vi "SRV_Read Motors Config File.vi"(0 "Motors Config File Path":path, 11 "error in (no error)":errorcluster) -> (4 "Motors Config File Path out":path, 8 "Motor Control Config":T1[](array[typedef]) {"Release Cmds"."Motor Control Commands Array"."Value" format="%02x"; "Release Cmds"."Motor Control Commands Array"."Register" format="%02x"; "Release Cmds"."Motor Control Commands Array"."I2C Address" format="%02x"; "Press Cmds"."Motor Control Commands Array"."Value" format="%02x"; "Press Cmds"."Motor Control Commands Array"."Register" format="%02x"; "Press Cmds"."Motor Control Commands Array"."I2C Address" format="%02x"}, 10 "Cancelled?":bool, 15 "error out":errorcluster)   [LabVIEW 2014]
doc: "Author: Mike Schultz (LogicPD, Inc)"
uses:
  SRV_Motor Control Button Config.ctl
  SRV_Motor Legos-Servo.ctl
  SRV_Motor Control Commands Cluster.ctl
  SRV_Motor Control Command Config.ctl
  SRV_Motor Control Button Icons_FALSE.ctl
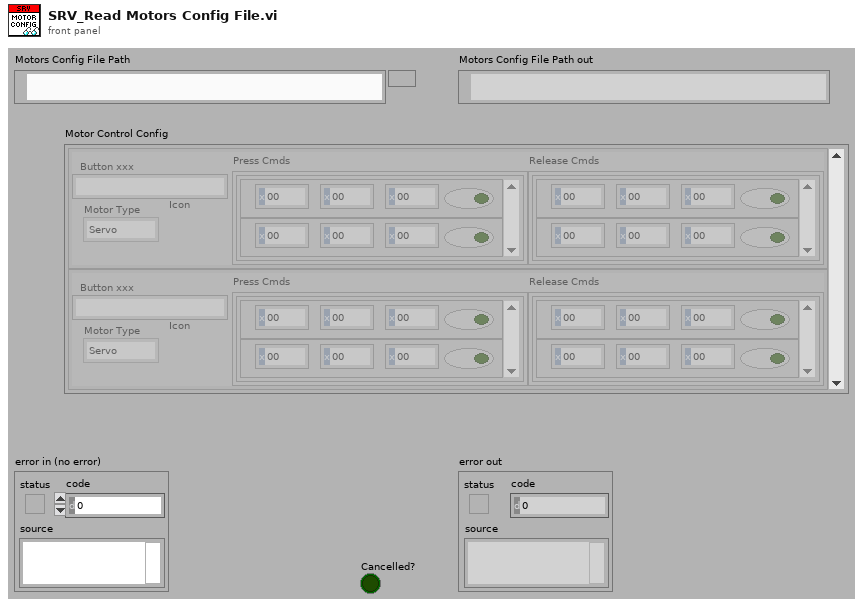
[diagram p1: front panel]
types:
  T1 = typedef "SRV_Motor Control Button Config.ctl" = cluster{"Button Name":string, "Button Label":string, "Motor Type":T2, "Press Cmds":T3, "Release Cmds":T3, "Icon":T5}
  T2 = typedef "SRV_Motor Legos-Servo.ctl" = enum16{"Servo", "Legos", "Shared Var"}
  T3 = typedef "SRV_Motor Control Commands Cluster.ctl" = cluster{"Motor Control Commands Array":T4[]}
  T4 = typedef "SRV_Motor Control Command Config.ctl" = cluster{"I2C Address":u8, "Register":u8, "Value":u8, "Active":bool}
  T5 = typedef "SRV_Motor Control Button Icons_FALSE.ctl" = u16
  T6 = enum16{"open", "open or create", "create or replace", "create", "open (read only)"}
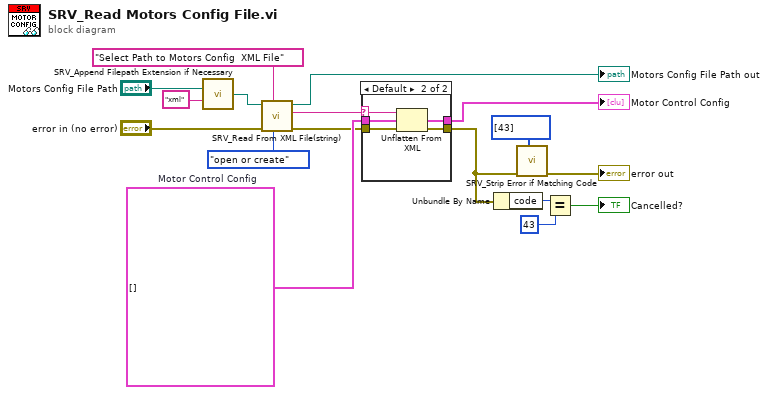
[diagram p0: block diagram]
diagram:
  w17 = T1[] []  # Motor Control Config
  n1 = call "SRV_Append Filepath Extension if Necessary.vi"("Filepath"="Motors Config File Path", "Extension"="xml") -> ("Filepath with Extension"=w11:path)  [unwired: 13 in]
  n2 = call "SRV_Read From XML File(string).vi"("function (open-read-only:4)"=T6."open or create", "Prompt"="Select Path to Motors Config  XML File", "error in (no error)"="error in (no error)", "XML File Path"=w11) -> ("error out"=w13:errorcluster, "XML Elements"=w9:string, "XML File Path(duplicate)"=→"Motors Config File Path out":path)  [unwired: 5 in]
  n3 = case shown="Default" w9 {
    selector: w9 -> [_ w20]
    tunnel: w17 -> [w18 w24]
    tunnel: [w18 w23] -> w7
    tunnel: [w19 w22] -> w2
    tunnel: w13 -> [w19 w21]
    frame "" {
    }
    frame Default {
      n4 = Unflatten From XML(xml string=w20, type=w24, error in (no error)=w21) -> (value=w23:T1[], error out=w22:errorcluster)
    }
  }
  "Motor Control Config" <- w7
  n5 = Unbundle By Name(w2) -> ("code"=w6:i32)
  n6 = call "SRV_Strip Error if Matching Code.vi"("error in (no error)"=w2, "Strip Codes"=i32[] [43]) -> ("error out"=→"error out":errorcluster)  [unwired: 8 in]
  n7 = Equal?(x=w6, y=43) -> (x = y?=→"Cancelled?":bool)
